vi "Configure Decision Feedback Equalization Taps.vi"(8 "error in (no error)":errorcluster, 10 "DFE Taps":dbl[](array[numeric]), 11 "VISA resource name":refnum<visa-resource-name>) -> (0 "error out":errorcluster, 3 "VISA resource name out":refnum<visa-resource-name>)   [LabVIEW 2020, in "Agilent 90000 Series.lvlib"]
doc: "Configures the taps for Decision Feedback Equalization."
uses:
  Agilent 90000 Series.lvlib
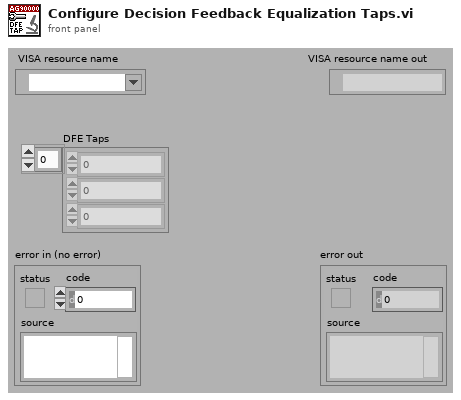
[diagram p1: front panel]
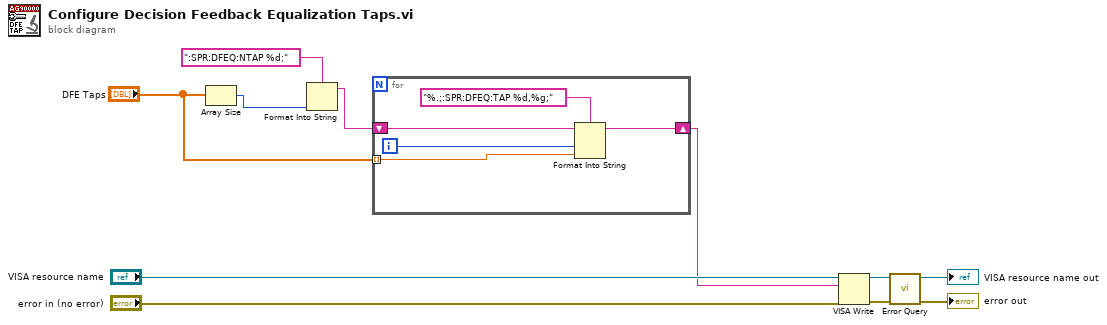
[diagram p0: block diagram]
diagram:
  n1 = Array Size(array="DFE Taps") -> (size(s)=w4:i32)
  n2 = Format Into String(format string=":SPR:DFEQ:NTAP %d;", w4) -> (resulting string=w2:string)  [unwired: 2 in, 1 out]
  n3 = for {
    tunnel: "DFE Taps" -> [w14] mode=indexing
    shift-right: [w12] -> w1
    shift-left: w2 -> [w13]
    i -> [w15]
    n4 = Format Into String(format string="%.;:SPR:DFEQ:TAP %d,%g;", initial string=w13, w15, w14) -> (resulting string=w12:string)  [unwired: 1 in, 1 out]
  }
  n5 = VISA Write(VISA resource name="VISA resource name", write buffer=w1, error in (no error)="error in (no error)") -> (VISA resource name out=w9:refnum<visa-resource-name>, error out=w8:errorcluster)  [unwired: 1 out]
  n6 = call "Error Query.vi"("error in (no error)"=w8, "VISA resource name"=w9) -> ("error out"=→"error out":errorcluster, "VISA resource name out"=→"VISA resource name out":refnum<visa-resource-name>)  [unwired: 8 out]
